vi "Read_WIP.vi"(8 "error in (no error)":errorcluster, 11 "Refnum in":T3) -> (0 "error out":errorcluster, 2 "WIP Limit":T1, 3 "Refnum out":T3)   [LabVIEW 2020]
uses:
  <vilib>/addons/database/Connection.llb/Conn ObjectReference.ctl
  Controls/WIP Limit.ctl
  Controls/WIP_old.ctl
  MS SQL/MS_Global.vi
  <vilib>/addons/database/_DB Variant To Data/Database Variant To Data.xnode
  <vilib>/addons/database/NI_Database_API.lvlib
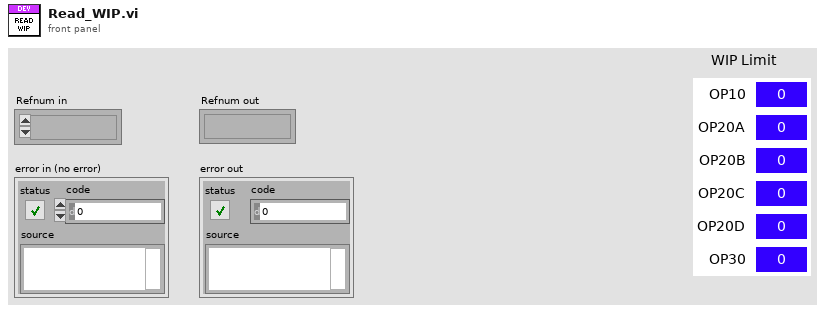
[diagram p1: front panel]
types:
  T1 = typedef "WIP Limit.ctl" = cluster{"OP10":T2, "OP20A":T2, "OP20B":T2, "OP20C":T2, "OP20D":T2, "OP30":T2}
  T2 = typedef "WIP_old.ctl" = i64
  T3 = typedef "NI_Database_API.lvlib/Conn ObjectReference.ctl" = refnum<k1>
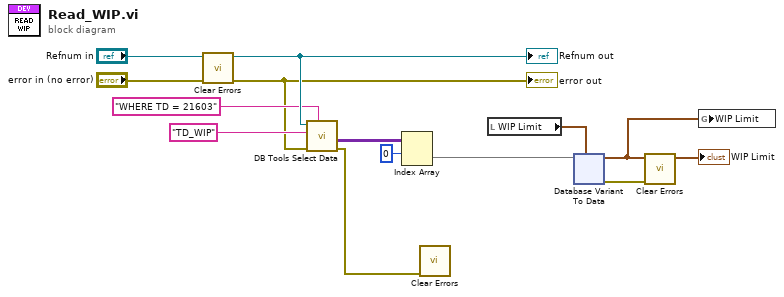
[diagram p0: block diagram]
diagram:
  n1 = call <vilib>:"Clear Errors.vi"("error in (no error)"="error in (no error)") -> ("error out"=w1:errorcluster)  [unwired: 5 in, 1 out]
  "error out" <- w1
  n2 = call <vilib>:"DB Tools Select Data.vi"("condition"="WHERE TD = 21603", "error in (no error)"=w1, "table"="TD_WIP", "connection reference"="Refnum in") -> ("error out"=w2:errorcluster, "data"=w9:variant[][])  [unwired: 2 in, 1 out]
  n3 = Index Array(array=w9, index (row)=0) -> (element=w6:variant[])  [unwired: 1 in]
  n4 = call <vilib>:"Clear Errors.vi"("error in (no error)"=w2) -> ()  [unwired: 5 in, 2 out]
  n5 = local read "WIP Limit"() -> (w5:T1)
  n6 = xnode "Database Variant To Data"("database variant"=w6, "type"=w5) -> ("data"=w3:T1, "error out"=w4:errorcluster)  [unwired: 1 in]
  "WIP Limit" <- w3
  n7 = call <vilib>:"Clear Errors.vi"("error in (no error)"=w4) -> ()  [unwired: 5 in, 2 out]
  n8 = global write "MS_Global.vi" "WIP Limit"(w3) -> ()
  "Refnum out" <- "Refnum in"
